vi "Sys config window-Save HW config.vi"(11 "Initial Configuration":T1={"System Config out"={"XY Stage"={"COM port"="", "XY stage available"=FALSE}, "DAQ FPGA"={"Ref"=refnum, "Target"="RIO0", "Clock Freq (MHz) "=200.0, "input card type"=enum."AC Card", "Samples Wait after Trigger"=5080, "AOD fill"=4900, "StartupDelay"=0, "Slip Cycle (clock cycles)"=600000, "Add Cycle"=TRUE}, "Control system"={"Ethernet opened"=FALSE, "Ethernet Port"=3, "Ctrl FPGA available"=FALSE, "Ctrl FPGA Clock (MHz)"=240.0, "Ctrl system MAC address"="", "Control system.Network adapter name"="", "AOD 1 Amplitude"=0, "AOD 2 Amplitude"=0, "AOD 3 Amplitude"=0, "AOD 4 Amplitude"=0, "Data Time Interval (ns)"=0.0, "T0 (ns)"=0.0, "Ta (ns)"=0.0}, "Encoder"={"IP address"="224.0.1.103", "Port"=7000, "Encoder available"=FALSE, "Wheel radius (cm)"=16.0}, "DAQmx Chan"={"Pockels AO"="", "Hard shutter AO"="", "PMT AOs"="", "Power meter AI"=""}, "Computer MAC address"="", "Cam VidRec"={"DO flag-Video record"="", "DO flag-Trial start"="", "VidRec available"=FALSE}, "Externalise Triggers"=FALSE, "Laser wavelength (nm)"=920.0}, "Triggers output setup"=[], "AOL Properties"={"AOD 1 thickness (mm)"=118.0, "AOD 2 thickness (mm)"=115.0, "AOD 3 thickness (mm)"=110.0, "AOD 4 thickness (mm)"=135.0, "AOD 1-2 separation (mm)"=135.0, "AOD 2-3 separation (mm)"=135.0, "AOD 3-4 separation (mm)"=15.0, "AOL aperture (mm)"=15.0, "AOL centre wavelength (nm)"=15.0, "AOL centre frequency (MHz)"=15.0, "skewZX"=15.0, "skewZY"=15.0, "magZX"=50.0, "magZY"=50.0, "Diffraction mode"=50.0, "Crystal length (mm)"=15.0, "Acoustic velocity (m/s)"=1.0, "Pair deflection ratio"=1.0, "AOD fill time (us)"=1.0}, "Calibration settings"={"Pockels cal.Zoom"=0, "Pockels cal.Dwell time (µs)"=0.0}} {"System Config out"."Laser wavelength (nm)" min=800.0 max=1080.0 step=1.0; "System Config out"."Encoder"."Wheel radius (cm)" format="%#_13g"; "System Config out"."Control system"."Ctrl FPGA Clock (MHz)" min=80.0 max=500.0 step=1.0; "System Config out"."Control system"."Data Time Interval (ns)" min=0.0 max=2048.0 step=1.0; "System Config out"."Control system"."Ta (ns)" min=0.0 max=2048.0 step=1.0; "System Config out"."Control system"."T0 (ns)" min=0.0 max=2048.0 step=1.0; "System Config out"."Control system"."AOD 4 Amplitude" min=0 max=2048 step=1; "System Config out"."Control system"."AOD 3 Amplitude" min=0 max=2048 step=1; "System Config out"."Control system"."AOD 2 Amplitude" min=0 max=2048 step=1; "System Config out"."Control system"."AOD 1 Amplitude" min=0 max=2048 step=1; "Triggers output setup"."Pulse width (us)" min=10 max=5000 step=1 format="%.0fµs"}) -> ()   [LabVIEW 2013]
uses:
  Configuration code/Typedefs/Initial config.ctl
  Typedefs/Sys Configuration.ctl
  Typedefs/XY Stage config cluster.ctl
  Typedefs/DAQ FPGA config cluster.ctl
  RIG-SPECIFIC FILES/FPGA Refs/FPGA Ref.ctl
  <vilib>/userdefined/High Color/nirio_resource_hc.ctl
  Typedefs/FPGA input type AC-DC.ctl
  Typedefs/CTRL system config cluster.ctl
  Typedefs/Encoder config cluster.ctl
  Typedefs/DAQmx physical channels cluster.ctl
  Typedefs/Cam VidRec HW config setup cluster.ctl
  Peripherals Control/Triggers/Typedefs/Triggers output setup.ctl
  Peripherals Control/Triggers/Typedefs/Trigger setup element cluster.ctl
  Typedefs/AOL Properties Cluster.ctl
  Configuration code/Typedefs/Calibration settings cluster.ctl
  Typedefs/Save-Load enum.ctl
  Typedefs/HW config states enum.ctl
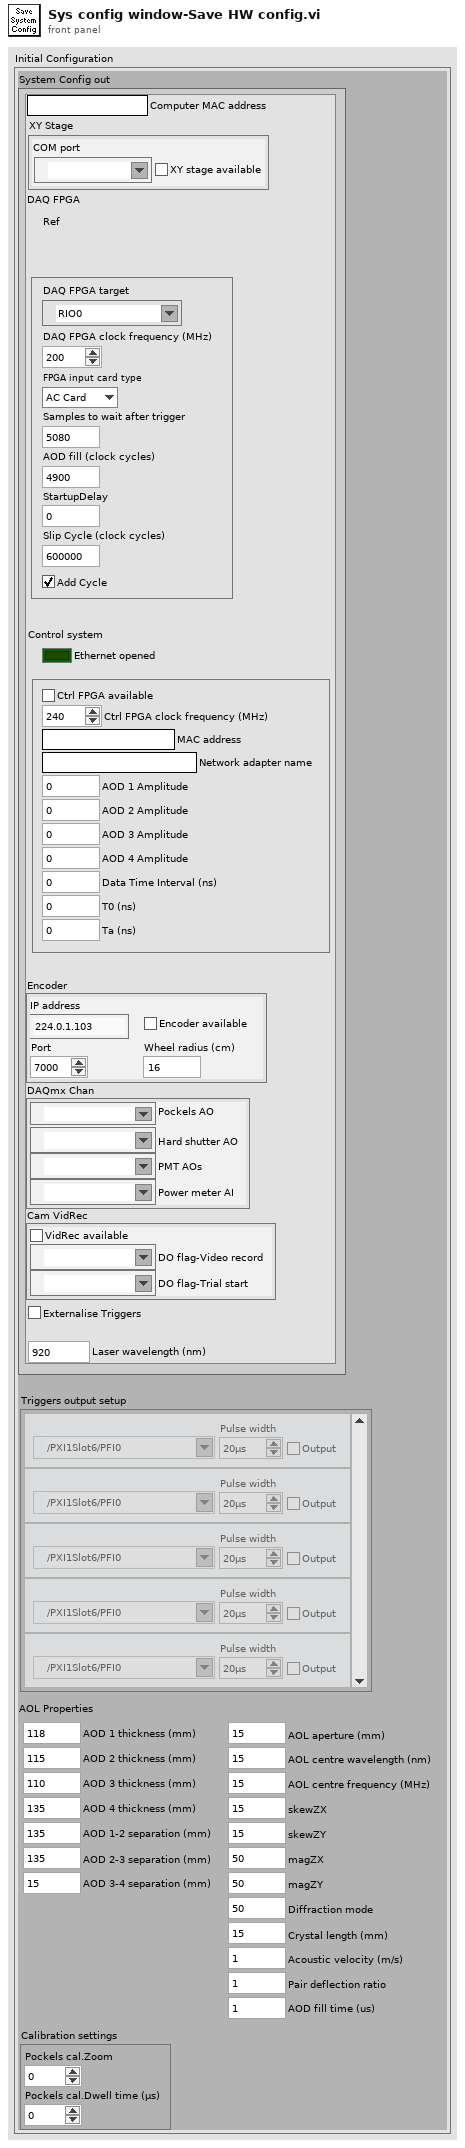
[diagram p1: front panel]
types:
  T1 = typedef "Initial config.ctl" = cluster{"System Config out":T2, "Triggers output setup":T12, "AOL Properties":T14, "Calibration settings":T15}
  T2 = typedef "Sys Configuration.ctl" = cluster{"XY Stage":T3, "DAQ FPGA":T4, "Control system":T8, "Encoder":T9, "DAQmx Chan":T10, "Computer MAC address":string, "Cam VidRec":T11, "Externalise Triggers":bool, "Laser wavelength (nm)":dbl}
  T3 = typedef "XY Stage config cluster.ctl" = cluster{"COM port":refnum<visa-resource-name>, "XY stage available":bool}
  T4 = typedef "DAQ FPGA config cluster.ctl" = cluster{"Ref":T5, "Target":T6, "Clock Freq (MHz) ":dbl, "input card type":T7, "Samples Wait after Trigger":u16, "AOD fill":u16, "StartupDelay":i32, "Slip Cycle (clock cycles)":u32, "Add Cycle":bool}
  T5 = typedef "FPGA Ref.ctl" = refnum<k20>
  T6 = typedef "nirio_resource_hc.ctl" = tag
  T7 = typedef "FPGA input type AC-DC.ctl" = enum16{"AC Card", "DC Card"}
  T8 = typedef "CTRL system config cluster.ctl" = cluster{"Ethernet opened":bool, "Ethernet Port":u32, "Ctrl FPGA available":bool, "Ctrl FPGA Clock (MHz)":dbl, "Ctrl system MAC address":string, "Control system.Network adapter name":string, "AOD 1 Amplitude":i16, "AOD 2 Amplitude":i16, "AOD 3 Amplitude":i16, "AOD 4 Amplitude":i16, "Data Time Interval (ns)":dbl, "T0 (ns)":dbl, "Ta (ns)":dbl}
  T9 = typedef "Encoder config cluster.ctl" = cluster{"IP address":string, "Port":u16, "Encoder available":bool, "Wheel radius (cm)":dbl}
  T10 = typedef "DAQmx physical channels cluster.ctl" = cluster{"Pockels AO":tag, "Hard shutter AO":tag, "PMT AOs":tag, "Power meter AI":tag}
  T11 = typedef "Cam VidRec HW config setup cluster.ctl" = cluster{"DO flag-Video record":tag, "DO flag-Trial start":tag, "VidRec available":bool}
  T12 = typedef "Triggers output setup.ctl" = T13[]
  T13 = typedef "Trigger setup element cluster.ctl" = cluster{"Name":string, "Output?":bool, "Output terminal":tag, "PXI backplane line":tag, "Pulse width (us)":u16}
  T14 = typedef "AOL Properties Cluster.ctl" = cluster{"AOD 1 thickness (mm)":dbl, "AOD 2 thickness (mm)":dbl, "AOD 3 thickness (mm)":dbl, "AOD 4 thickness (mm)":dbl, "AOD 1-2 separation (mm)":dbl, "AOD 2-3 separation (mm)":dbl, "AOD 3-4 separation (mm)":dbl, "AOL aperture (mm)":dbl, "AOL centre wavelength (nm)":dbl, "AOL centre frequency (MHz)":dbl, "skewZX":dbl, "skewZY":dbl, "magZX":dbl, "magZY":dbl, "Diffraction mode":dbl, "Crystal length (mm)":dbl, "Acoustic velocity (m/s)":dbl, "Pair deflection ratio":dbl, "AOD fill time (us)":dbl}
  T15 = typedef "Calibration settings cluster.ctl" = cluster{"Pockels cal.Zoom":u8, "Pockels cal.Dwell time (µs)":dbl}
  T16 = typedef "HW config states enum.ctl" = enum16{"Load from file", "Save to file", "Write all", "Read all", "Write XY stage settings", "Write DAQ FPGA settings", "Write Control FPGA settings", "Write Phys Channels", "Clear", "Compare from file"}
  T17 = typedef "Save-Load enum.ctl" = enum16{"Save to file", "Load from file", "Compare from file"}
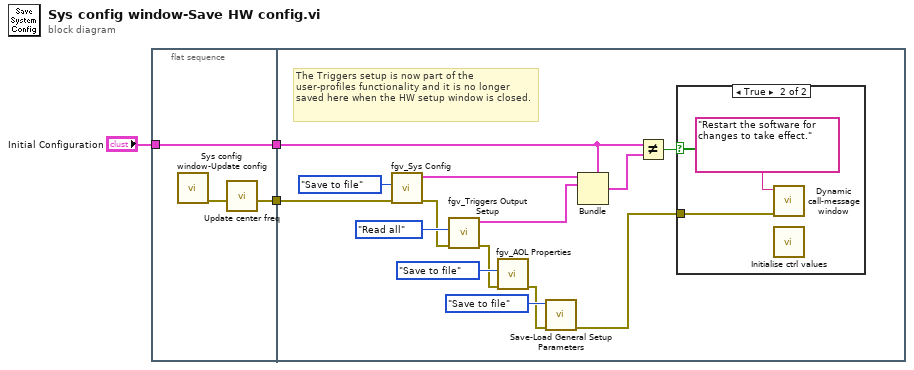
[diagram p0: block diagram]
diagram:
  n1 = flat-sequence {
    tunnel: "Initial Configuration" -> [w6]
    tunnel: [w6] -> w2
    tunnel: [w4] -> w1
    tunnel: w2 -> [w19]
    tunnel: w1 -> [w13]
    frame #0 {
      n2 = call "Sys config window-Update config.vi"() -> ("error out"=w5:errorcluster)  [unwired: 11 in]
      n3 = call "Update center freq.vi"("error in (no error)"=w5) -> ("error out"=w4:errorcluster)  [unwired: 10 in]
    }
    frame #1 {
      # "The Triggers setup is now part of the user-profiles functionality and it is no longer saved here when the HW setup window is closed."
      n4 = call "fgv_Sys Config.vi"("error in (no error)"=w13, "Function"=HW_config_states_enum."Save to file") -> ("error out"=w10:errorcluster, "System Config out"=w18:T2)  [unwired: 8 in]
      n5 = call "fgv_Triggers Output Setup.vi"("error in (no error)"=w10, "Function"=HW_config_states_enum."Read all") -> ("error out"=w9:errorcluster, "Triggers output setup"=w17:T12)  [unwired: 8 in]
      n6 = call "fgv_AOL Properties.vi"("error in (no error)"=w9, "Function"=HW_config_states_enum."Save to file") -> ("error out"=w8:errorcluster)  [unwired: 8 in, 1 out]
      n7 = call "Save-Load General Setup Parameters.vi"("error in"=w8, "Function"=Save-Load_enum."Save to file") -> ("error out"=w7:errorcluster)  [unwired: 9 in]
      n8 = Bundle(cluster=w19, "System Config out"=w18, "Triggers output setup"=w17) -> (w16:T1)  [unwired: 2 in]
      n9 = Not Equal?(x=w19, y=w16) -> (x != y?=w20:bool)
      n10 = case shown="True" w20 {
        tunnel: w7 -> [_ w22]
        frame False {
        }
        frame True {
          n11 = call "Dynamic call-message window.vi"("error in (no error)"=w22, "Message"="Restart the software for changes to take effect.") -> ()  [unwired: 9 in, 1 out]
          n12 = call "Initialise ctrl values.vi"() -> ()  [unwired: 11 in, 1 out]
        }
      }
    }
  }
